vi "FormatMechanicalAction.vi"(1 "mechanical action":T1=enum."LATCH_UNTIL_RELEASED") -> (0 "value":string)   [LabVIEW 2014, in "Raspberry Pi Compatible Compiler for LabVIEW.lvlib" / "PythonConfiguration.lvclass"]
uses:
  PythonConfiguration.lvclass
  TypeDefs/MechanicalActionTD.ctl
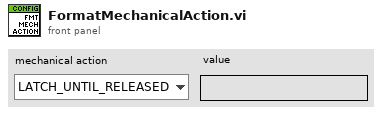
[diagram p1: front panel]
types:
  T1 = typedef "Raspberry Pi Compatible Compiler for LabVIEW.lvlib/PythonConfiguration.lvclass/MechanicalActionTD.ctl" = enum32{"SWITCH_WHEN_PRESSED", "SWITCH_WHEN_RELEASED", "SWITCH_UNTIL_RELEASED", "LATCH_WHEN_PRESSED", "LATCH_WHEN_RELEASED", "LATCH_UNTIL_RELEASED"}
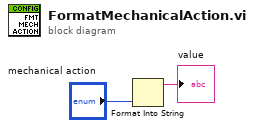
[diagram p0: block diagram]
diagram:
  n1 = Format Into String("mechanical action") -> (resulting string=→"value":string)  [unwired: 3 in, 1 out]
